vi "Truly_Arbitrary_Waveform Generator.vi"() -> ()   [LabVIEW 2020]
panel:
  in  "Phase (0-2pi)":dbl[](array[slide]) scale=0.0..6.28
  in  "Amplitude (1/x)":dbl[][](array[numeric]) min=0.0 max=50.0
  in  "stop":bool
  in  "Amplitude":dbl=0.7 format="%#_13g"
  in  "Frequency  (Hz)":i32=4000
  in  "Channel":i32(ring)=1 items=["Channel 1"=1, "Channel 2"=2]
  in  "Start":bool
  out "Waveform Graph 1":dbl[](graph)
  in  "IP address":string="192.168.1.100"
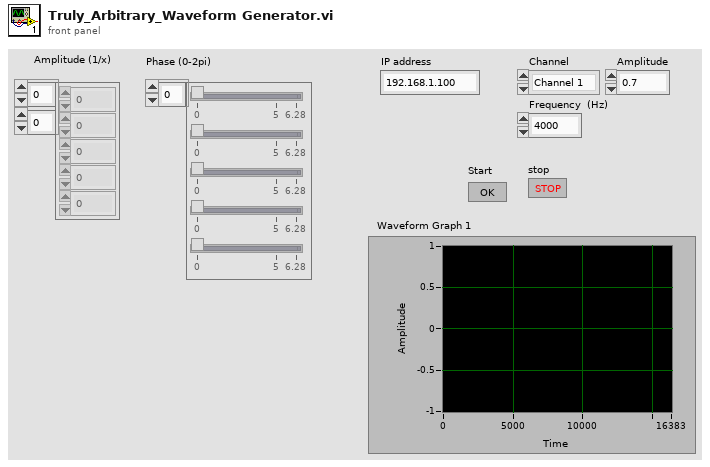
[diagram p1: front panel]
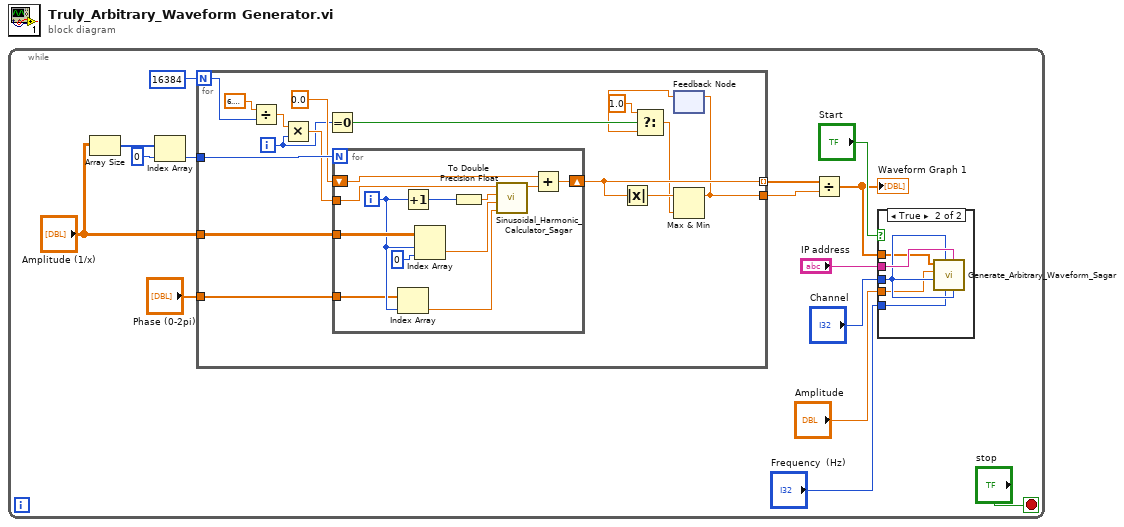
[diagram p0: block diagram]
diagram:
  n1 = while {
    stop <- "stop" stop-if-true
    n2 = Array Size(array="Amplitude (1/x)") -> (size(s)=w8:i32[])
    n3 = Index Array(array=w8, index=0) -> (element=w5:i32)
    n4 = for {
      N: 16384 -> [w22]
      tunnel: w5 -> [w29]
      tunnel: "Amplitude (1/x)" -> [w26]
      tunnel: [w24] -> w3 mode=indexing
      tunnel: "Phase (0-2pi)" -> [w25]
      tunnel: [w16] -> w1
      i -> [w18]
      n5 = Divide(x=6.283185307179586, y=w22) -> (x/y=w30:dbl)
      n6 = Multiply(x=w30, y=w18) -> (x*y=w28:dbl)
      n7 = Equal To 0?(x=w18) -> (x = 0?=w21:bool)
      n8 = for {
        N: w29 -> [_]
        tunnel: w28 -> [w43]
        shift-right: [w41] -> w24
        shift-left: 0.0 -> [w42]
        tunnel: w26 -> [w39]
        tunnel: w25 -> [w33]
        i -> [w34]
        n9 = Index Array(array=w33, index=w34) -> (element=w32:dbl)
        n10 = Increment(x=w34) -> (x+1=w37:i32)
        n11 = Index Array(array=w39, index (row)=w34, index (col)=0 ("disabled index (col)")) -> (element=w35:dbl)
        n12 = To Double Precision Float(number=w37) -> (double precision float=w36:dbl)
        n13 = call "Sinusoidal_Harmonic_Calculator_Sagar.vi"("Phase"=w32, "Amplitude (1/x)"=w35, "Harmonic"=w36, "Numeric in"=w43) -> ("Numeric out"=w40:dbl)  [unwired: 7 in]
        n14 = Add(x=w42, y=w40) -> (x+y=w41:dbl)
      }
      n15 = Absolute Value(x=w24) -> (abs(x)=w23:dbl)
      n16 = feedback #1() -> (w20:dbl)  [unwired: 1 in]
      n17 = Select(t=1.0, s=w21, f=w20) -> (s? t:f=w17:dbl)
      n18 = Max & Min(x=w23, y=w17) -> (max(x,y)=w16:dbl)  [unwired: 1 out]
      n19 = feedback-in #1(w16) -> ()
    }
    n20 = Divide(x=w3, y=w1) -> (x/y=w2:dbl[])
    "Waveform Graph 1" <- w2
    n21 = case shown="True" "Start" {
      tunnel: "IP address" -> [_ w48]
      tunnel: "Channel" -> [_ w47]
      tunnel: "Frequency  (Hz)" -> [_ w46]
      tunnel: "Amplitude" -> [_ w45]
      tunnel: w2 -> [_ w44]
      frame False {
      }
      frame True {
        n22 = call "Generate_Arbitrary_Waveform_Sagar.vi"("Channel (1|2)"=w47, "IP address"=w48, "Frequency (1000 Hz)"=w46, "Channel (0: 1)"=w47, "Channel (1|2) 2"=w47, "Amplitude"=w45, "Array"=w44) -> ()  [unwired: 5 in]
      }
    }
  }
